vi "Person Custom Probe.vi"(11 "Person out":refnum<class "Person.lvclass">) -> (2 "Value String":string, 3 "Boolean":bool)   [LabVIEW 2017, in "Person.lvclass"]
uses:
  Person.lvclass
  Person.lvclass/Person.ctl
  Get firstName.vi
  Get lastName.vi
  Get Age.vi
panel:
  out "resulting string":string
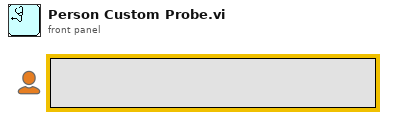
[diagram p1: front panel]
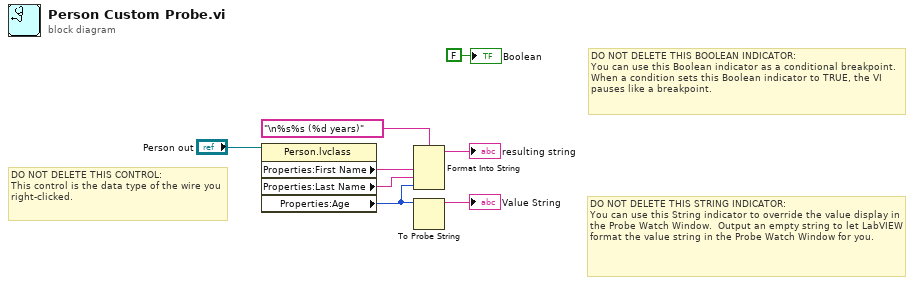
[diagram p0: block diagram]
diagram:
  # "DO NOT DELETE THIS STRING INDICATOR: \nYou can use this String indicator to override the value display in the Probe Watch Window.  Output an empty string to let LabVIEW format the value string in the Probe Watch Window for you."
  # "DO NOT DELETE THIS BOOLEAN INDICATOR: \nYou can use this Boolean indicator as a conditional breakpoint. When a condition sets this Boolean indicator to TRUE, the VI pauses like a breakpoint."
  # "DO NOT DELETE THIS CONTROL: \nThis control is the data type of the wire you right-clicked."
  n1 = property class="Person.lvclass"(reference="Person out") -> ("Properties:First Name"=w7:string, "Properties:Last Name"=w6:string, "Properties:Age"=w2:i32)  [unwired: 1 in, 2 out]
  n2 = Format Into String(format string="\n%s%s (%d years)", w7, w6, w2) -> (resulting string=→"resulting string":string)  [unwired: 2 in, 1 out]
  n3 = To Probe String(7:w2) -> (3:→"Value String":string)  [unwired: 2 in, 1 out]
  "Boolean" <- FALSE ("Boolean")
